vi "System Monitor Example.vi"() -> ()   [LabVIEW 2014]
panel:
  out "Mem  Chart":dbl(graph)
  out "Mem Usage":string
  out "Mem Usage":dbl(slide) scale=0.0..100.0 scale format="%_1f"
  out "CPU Chart":dbl(graph)
  out "CPU Usage":string
  out "CPU Usage":dbl(slide) scale=0.0..100.0 scale format="%_1f"
  in  "stop":bool
  out "Status":string
  # "CPU Usage"
  # "CPU Usage History"
  # "Available Mem"
  # "Available Memory History"
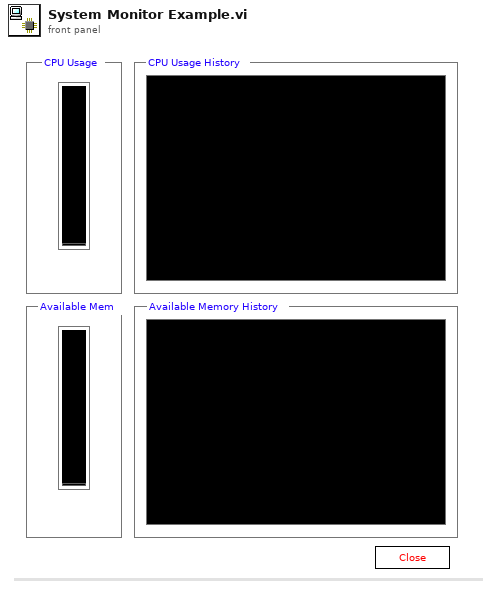
[diagram p1: front panel]
types:
  T1 = typedef "tools_windows CPU Usage Ref.ctl" = cluster{"Query":u32, "Counter":u32}
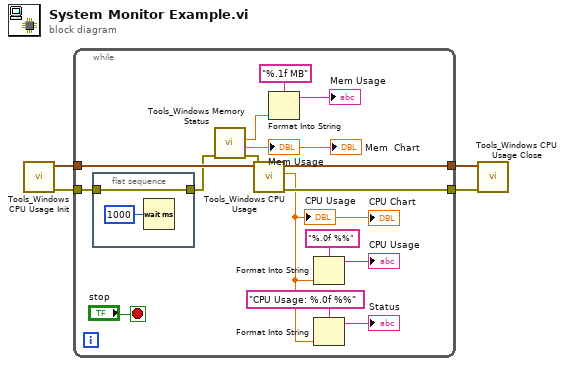
[diagram p0: block diagram]
diagram:
  n1 = call "Tools_Windows CPU Usage Init.vi"() -> ("error out"=w1:errorcluster, "CPU Usage Ref"=w3:T1)  [unwired: 10 in]
  n2 = while {
    tunnel: [w20] -> w4
    tunnel: w3 -> [w16]
    tunnel: [w15] -> w2
    tunnel: w1 -> [w14]
    stop <- "stop" stop-if-true
    n3 = flat-sequence {
      tunnel: w14 -> [w21]
      tunnel: [w21] -> w10
      frame #0 {
        n4 = Wait (ms)(milliseconds to wait=u32 1000) -> ()  [unwired: 1 out]
      }
    }
    n5 = call "Tools_Windows Memory Status.vi"("error in (no error)"=w10) -> ("error out"=w9:errorcluster, "Free memory (%)"=→"Mem Usage" →"Mem  Chart":dbl, "Free memory (KB)"=w5:dbl)  [unwired: 7 in, 1 out]
    n6 = call "Tools_Windows CPU Usage.vi"("error in"=w9, "CPU Usage Ref"=w16) -> ("error out"=w20:errorcluster, "CPU Usage (%)"=w13:dbl, "CPU Usage Ref"=w15:T1)  [unwired: 7 in]
    "CPU Usage" <- w13
    "CPU Chart" <- w13
    n7 = Format Into String(format string="%.1f MB", w5) -> (resulting string=→"Mem Usage":string)  [unwired: 2 in, 1 out]
    n8 = Format Into String(format string="%.0f %%", w13) -> (resulting string=→"CPU Usage":string)  [unwired: 2 in, 1 out]
    n9 = Format Into String(format string="CPU Usage: %.0f %%", w13) -> (resulting string=→"Status":string)  [unwired: 2 in, 1 out]
  }
  n10 = call "Tools_Windows CPU Usage Close.vi"("error in"=w4, "CPU Usage Ref"=w2) -> ()  [unwired: 9 in, 1 out]
